vi "CRYTS Sequence Insert.vi"(10 "Steps":refnum<vi>, 11 "Tree Task SequenceIn":refnum<vi>) -> (3 "Tree Task Sequence Out":refnum<vi>)   [LabVIEW 2013]
uses:
  CRYProject Editor Global.vi
  CRYMainGlobal.vi
  CRYCurveLibrary/Global/CRYCurve Library Global.vi
panel:
  # "Insert new step into Project window."
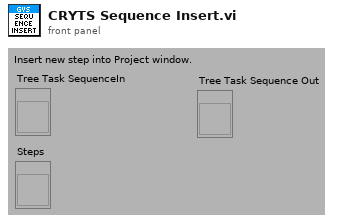
[diagram p1: front panel]
types:
  T1 = typedef "CRYTS.ctl" = cluster{"No.TS":u16, "TS File Path":path, "TS Name":string, "EditStepName":string, "Steps":T2[], "New State":bool, "Change State":bool, "Flattened CurveLib Data":string, "Document Data":string, "EditStepNo":u16, "Operator Start File":string, "Sequence Type":string, "Sequence Language":string}
  T2 = typedef "CRYStep.ctl" = cluster{"No.VI":i32, "Category":string, "StepName":string, "Seq setup flattened":string, "Comment":string, "Steps config.":bool[], "Jump config":i32[], "Start":dbl, "Increment":dbl, "Name":string, "Unit":string, "Y data":u16, "Y prefix":string, "Y dB ref":dbl, "Y unit":string, "Repeat State Array":cluster{"Start":dbl, "Increment":dbl, "Count":i32, "Num":i32}[]}
  T3 = typedef "CRYSequence Cluster.ctl" = cluster{"EditStepName":string, "Trimmed string array":string, "Flattened CurveData":string, "Document Data":string, "EditStepNo":u16, "Operator Start File":path, "Sequence Type":string, "Sequence Language":string, "Sequence Work State":string}
  T4 = cluster{"Data type":string, "Version":u16, "Dimensions":u8}
  T5 = enum32{"English", "Chinese", "Korean", "Japanese", "Russian", "Chinese traditional"}
  T6 = enum16{"OK", "Yes", "YesNo", "YesNoCancel", "ReplaceAppend"}
  T7 = enum16{"Insert", "Remove", "Move up", "Move down"}
  T8 = cluster{"Start":dbl, "Increment":dbl, "Count":i32, "Num":i32}[]
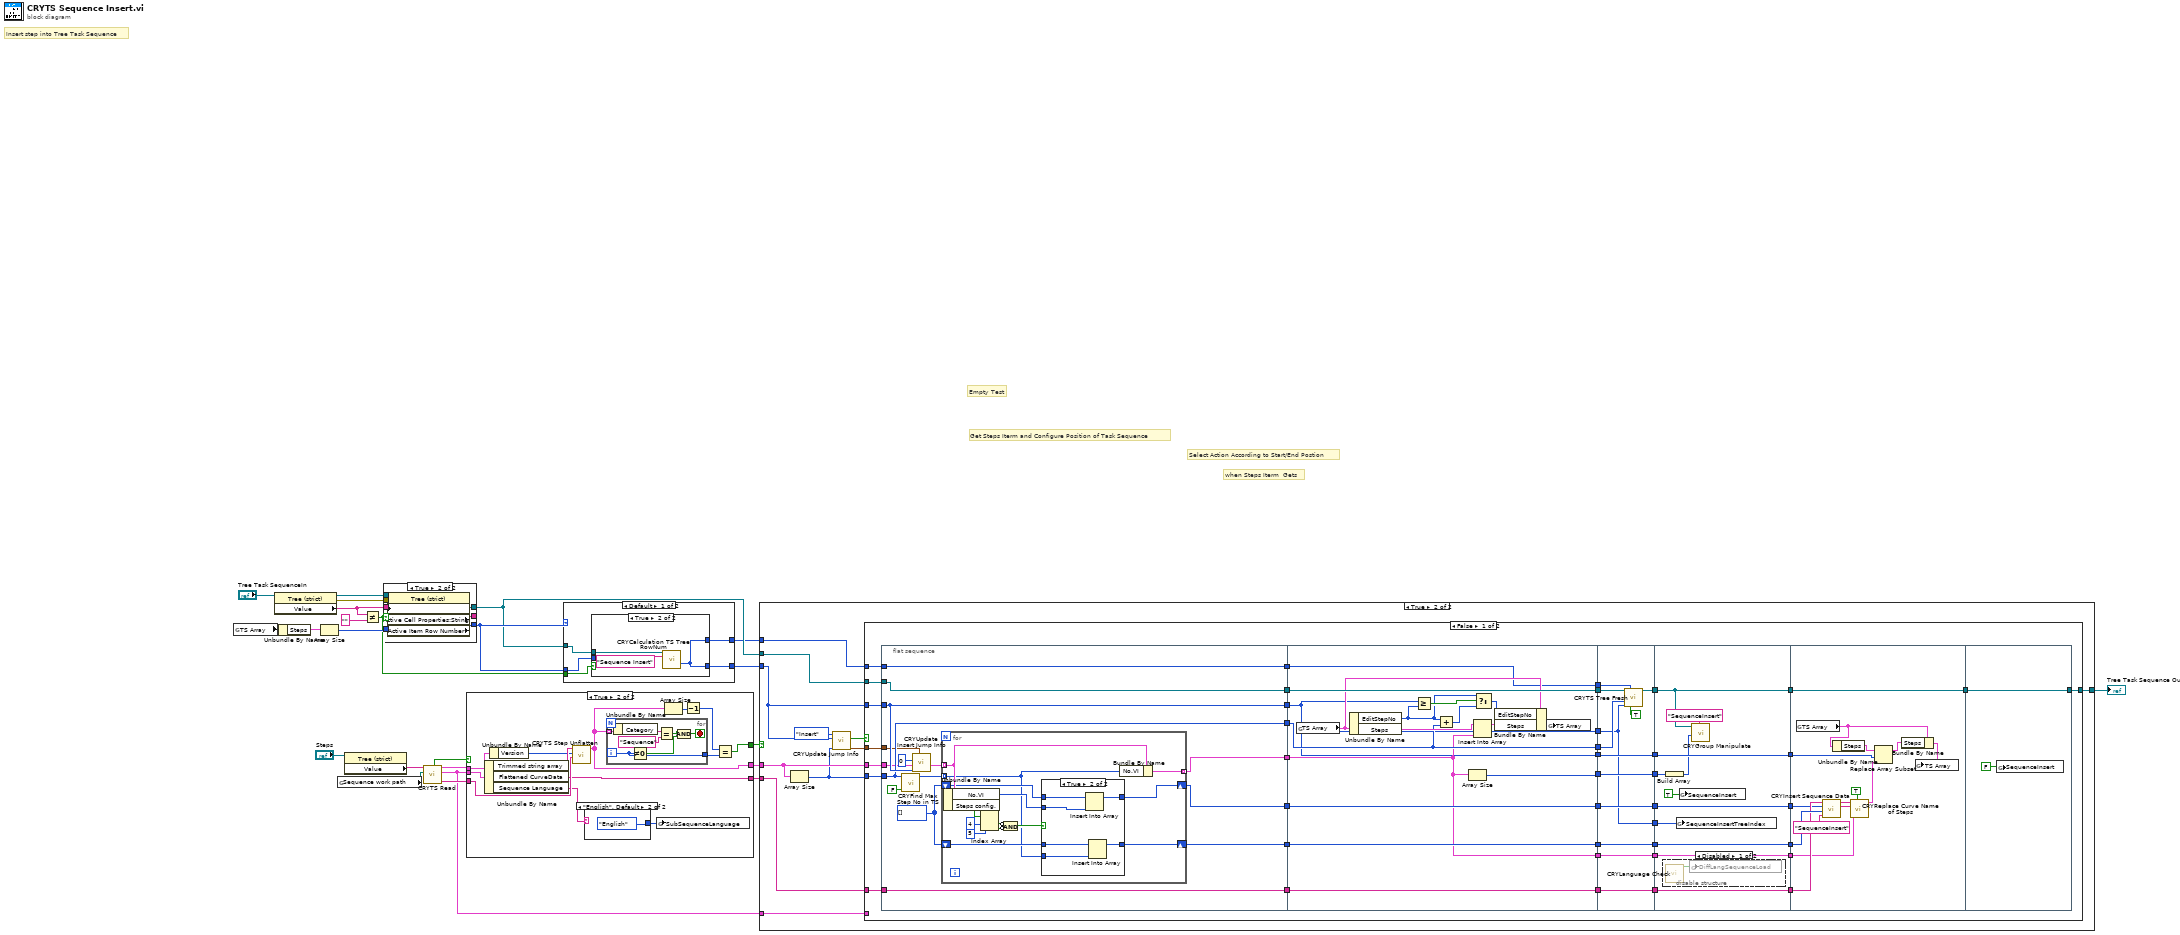
[diagram p0: block diagram]
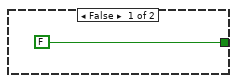
[diagram p2: hidden frame]
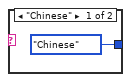
[diagram p3: hidden frame]
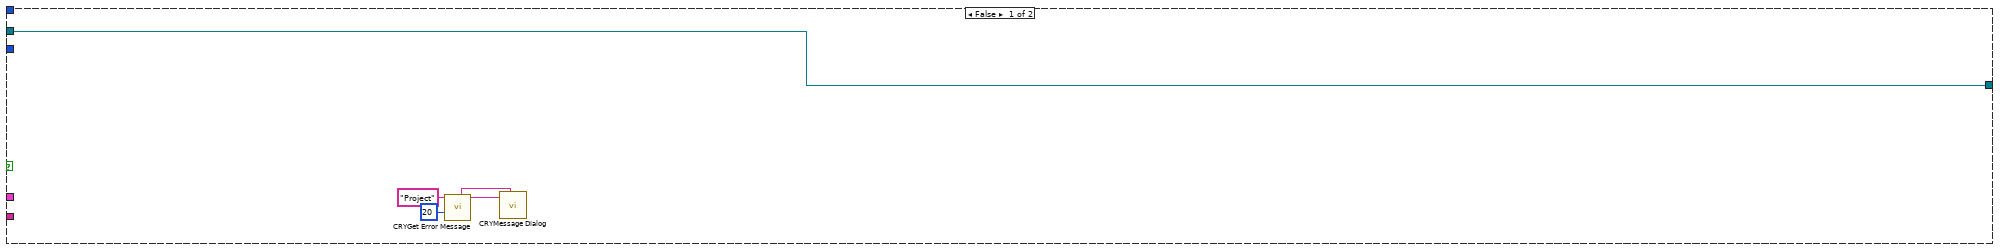
[diagram p4: hidden frame]
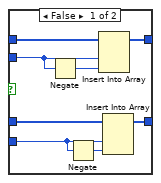
[diagram p5: hidden frame]
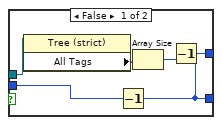
[diagram p8: hidden frame]
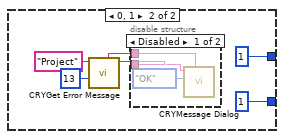
[diagram p9: hidden frame]
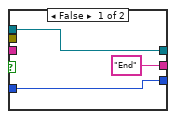
[diagram p11: hidden frame]
diagram:
  # "when Steps Iterm  Gets"
  # "Select Action According to Start/End Postion"
  # "Get Steps Iterm and Configure Position of Task Sequence"
  # "Empty Test"
  # "Insert step into Tree Task Sequence"
  n1 = global read "CRYProject Editor Global.vi" "TS Array"() -> (w22:T1)
  n2 = property class="Tree (strict)"(reference="Tree Task SequenceIn") -> (reference out=w18:refnum<vi>, error out=w17:errorcluster, "Value"=w16:string)  [unwired: 1 in]
  n3 = Unbundle By Name(w22) -> ("Steps"=w19:T2[])
  n4 = Array Size(array=w19) -> (size(s)=w14:i32)
  n5 = global read "CRYMainGlobal.vi" "Sequence work path"() -> (w9:path)
  n6 = property class="Tree (strict)"(reference="Steps") -> ("Value"=w20:string)  [unwired: 1 in, 2 out]
  n7 = Not Equal?(x=w16, y="") -> (x != y?=w6:bool)
  n8 = case shown="True" w6 {
    tunnel: w17 -> [_ w33]
    tunnel: ["End" ("Cell String") w32] -> _
    tunnel: [w25 w31] -> w7
    tunnel: [w27 w30] -> w5
    tunnel: w16 -> [_ w29]
    tunnel: w18 -> [w27 w28]
    tunnel: w14 -> [w25 _]
    frame False {
    }
    frame True {
      n9 = property class="Tree (strict)"(reference=w28, error in=w33, "Active Item Properties:Active Item (Tag)"=w29) -> (reference out=w30:refnum<vi>, "Active Cell Properties:String"=w32:string, "Active Item Row Number"=w31:i32)  [unwired: 1 out]
    }
  }
  n10 = call "CRYTS Read.vi"("Sequence folder path"=w9, "File Name"=w20) -> ("Sequence Name"=w12:string, "sequence list"=w1:T3, "Header info"=w10:T4, "status"=w11:bool)  [unwired: 6 out]
  n11 = case shown="True" w11 {
    tunnel: w1 -> [_ w47]
    tunnel: [FALSE ("status") w37] -> w8
    tunnel: w10 -> [_ w45]
    tunnel: w12 -> [_ w43]
    tunnel: [_ w38] -> w4
    tunnel: [_ w42] -> w3
    frame False {
    }
    frame True {
      n12 = Unbundle By Name(w47) -> ("Trimmed string array"=w46:string, "Flattened CurveData"=w42:string, "Sequence Language"=w35:string)
      n13 = Unbundle By Name(w45) -> ("Version"=w44:u16)
      n14 = call "CRYTS Step Unflatten.vi"("Sequence Name"=w43, "Version"=w44, "Flattened Steps"=w46) -> ("Unflattened Steps"=w38:T2[])  [unwired: 8 out]
      n15 = case shown="\"English\", Default" w35 {
        tunnel: [T5."Chinese" ("Language") T5."English" ("Language")] -> w36
        frame "Chinese" {
        }
        frame "English", Default {
        }
      }
      n16 = for {
        tunnel: w38 -> [w56] mode=indexing
        tunnel: [w50] -> w40
        i -> [w50]
        stop <- w51 stop-if-true
        n17 = Unbundle By Name(w56) -> ("Category"=w55:string)
        n18 = Not Equal To 0?(x=w50) -> (x != 0?=w52:bool)
        n19 = Equal?(x=w55, y="Sequence" ("x")) -> (x = y?=w53:bool)
        n20 = Compound Arithmetic op=AND(w53, w52) -> (w51:bool)
      }
      n21 = global write "CRYProject Editor Global.vi" "SubSequenceLanguage"(w36) -> ()
      n22 = Array Size(array=w38) -> (size(s)=w39:i32)
      n23 = Decrement(x=w39) -> (x-1=w41:i32)
      n24 = Equal?(x=w41, y=w40) -> (x = y?=w37:bool)
    }
  }
  n25 = case shown="Default" w7 {
    tunnel: w7 -> [w59 _]
    tunnel: [w58 1 ("Active Item Row Number")] -> w13
    tunnel: w6 -> [w61 _]
    tunnel: w5 -> [w60 _]
    tunnel: [w57 1 ("TargetRowNum")] -> w2
    frame Default {
      n26 = case shown="True" w61 {
        tunnel: w59 -> [w66 _]
        tunnel: [w62 w67] -> w58
        tunnel: w60 -> [w64 w69]
        tunnel: [w62 w67] -> w57
        frame False {
          n27 = property class="Tree (strict)"(reference=w64) -> ("All Tags"=w65:string[])  [unwired: 1 in, 2 out]
          n28 = Decrement(x=w66) -> (x-1=w62:i32)
          n29 = Array Size(array=w65) -> (size(s)=w63:i32)
          n30 = Decrement(x=w63) -> ()  [unwired: 1 out]
        }
        frame True {
          n31 = call "CRYCalculation TS Tree RowNum.vi"("Tree Task SequenceIn"=w69, "sOption"="Sequence Insert") -> ("TargetRowNum"=w67:i32)  [unwired: 7 in, 6 out]
        }
      }
    }
    frame 0, 1 {
      n32 = call "CRYGet Error Message.vi"("Error No"=13, "Kind"="Project") -> ("Message"=w72:string, "Window Title"=w71:string)  [unwired: 4 in, 4 out]
      n33 = disable-structure shown="Disabled" {
        disable-tunnel: w72 -> [w77 _]
        disable-tunnel: w71 -> [w76 _]
        frame Disabled {
          n34 = call "CRYMessage Dialog.vi"("Window Title"=w76, "YesNoCancel"=T6."OK", "Message Content"=w77) -> ()  [unwired: 7 in, 2 out]
        }
        frame Enabled {
        }
      }
    }
  }
  n35 = case shown="True" w8 {
    tunnel: [w83 w94] -> w24
    tunnel: w13 -> [_ w92]
    tunnel: w5 -> [w83 w93]
    tunnel: w4 -> [_ w90]
    tunnel: w3 -> [_ w87]
    tunnel: w2 -> [_ w86]
    tunnel: w1 -> [_ w84]
    frame False {
      n36 = call "CRYGet Error Message.vi"("Error No"=20, "Kind"="Project") -> ("Message"=w82:string, "Window Title"=w81:string)  [unwired: 4 in, 4 out]
      n37 = call "CRYMessage Dialog.vi"("Window Title"=w81, "Message Content"=w82) -> ()  [unwired: 8 in, 2 out]
    }
    frame True {
      n38 = Array Size(array=w90) -> (size(s)=w89:i32)
      n39 = call "CRYUpdate Jump Info.vi"("SourceCount"=w89, "Step number Selected"=w92, "Action"=T7."Insert") -> ("Jump State Out"=w85:T8, "Canceled?"=w91:bool)  [unwired: 7 in]
      n40 = case shown="False" w91 {
        tunnel: w92 -> [w135 _]
        tunnel: [w134 w237] -> w94
        tunnel: w90 -> [w133 _]
        tunnel: w89 -> [w132 _]
        tunnel: w93 -> [w131 w237]
        tunnel: w87 -> [w130 _]
        tunnel: w86 -> [w124 _]
        tunnel: w85 -> [w120 _]
        tunnel: w84 -> [_ _]
        frame False {
          n41 = flat-sequence {
            tunnel: [w148] -> w129
            tunnel: [w150] -> w128
            tunnel: [w149] -> w127
            tunnel: w130 -> [w137]
            tunnel: w131 -> [w148]
            tunnel: w132 -> [w149]
            tunnel: w133 -> [w147]
            tunnel: w135 -> [w150]
            tunnel: w124 -> [w141]
            tunnel: [w141] -> w123
            tunnel: w120 -> [w140]
            tunnel: [w139] -> w119
            tunnel: [w138] -> w116
            tunnel: [w137] -> w114
            tunnel: [w136] -> w112
            tunnel: w129 -> [w195]
            tunnel: w128 -> [w184]
            tunnel: w127 -> [w186]
            tunnel: [w195] -> w126
            tunnel: [w186] -> w125
            tunnel: w123 -> [w185]
            tunnel: [w185] -> w122
            tunnel: [w184] -> w121
            tunnel: w119 -> [w179]
            tunnel: [w184] -> w118
            tunnel: [w183] -> w117
            tunnel: w116 -> [w183]
            tunnel: [w182] -> w115
            tunnel: w114 -> [w182]
            tunnel: [w181] -> w113
            tunnel: w112 -> [w181]
            tunnel: [w180] -> w101
            tunnel: [w179] -> w97
            tunnel: w126 -> [w205]
            tunnel: w125 -> [w206]
            tunnel: w122 -> [w203]
            tunnel: w121 -> [w197]
            tunnel: [w204] -> w111
            tunnel: [w202] -> w109
            tunnel: w118 -> [w202]
            tunnel: [w201] -> w107
            tunnel: w117 -> [w201]
            tunnel: [w200] -> w105
            tunnel: w115 -> [w200]
            tunnel: [w199] -> w103
            tunnel: w113 -> [w199]
            tunnel: w101 -> [w198]
            tunnel: [w198] -> w100
            tunnel: [w197] -> w99
            tunnel: w97 -> [w196]
            tunnel: [w196] -> w96
            tunnel: w111 -> [w213]
            tunnel: [w213] -> w110
            tunnel: w109 -> [w218]
            tunnel: [w218] -> w108
            tunnel: w107 -> [w217]
            tunnel: [w217] -> w106
            tunnel: w105 -> [w216]
            tunnel: [w216] -> w104
            tunnel: w103 -> [w215]
            tunnel: [w215] -> w102
            tunnel: w100 -> [w212]
            tunnel: w99 -> [w209]
            tunnel: w96 -> [w208]
            tunnel: [w208] -> w95
            tunnel: w110 -> [w234]
            tunnel: w108 -> [w231]
            tunnel: w106 -> [w225]
            tunnel: w104 -> [w224]
            tunnel: w102 -> [w223]
            tunnel: [w234] -> w98
            tunnel: w95 -> [w220]
            tunnel: [w236] -> w134
            tunnel: w98 -> [w236]
            frame #0 {
              w143 = i32[] []
              n42 = call "CRYFind Max Step No in TS.vi"("Inputflg"=FALSE, "Required Count"=w149) -> ("Num Array Out"=w144:i32[])  [unwired: 1 in, 8 out]
              n43 = call "CRYUpdate Insert Jump Info.vi"("Jump State In"=w140, "Count"=w150, "Steps In"=w147, "Step number Selected"=0) -> ("Steps Out"=w145:T2[])  [unwired: 6 in, 1 out]
              n44 = for {
                tunnel: w145 -> [w163] mode=indexing
                tunnel: w144 -> [w151] mode=indexing
                tunnel: [w164] -> w139 mode=indexing
                shift-right: [w154] -> w136
                shift-left: w143 -> [w155]
                shift-right: [w152] -> w138
                shift-left: w143 -> [w153]
                n45 = Unbundle By Name(w163) -> ("No.VI"=w156:i32, "Steps config."=w162:bool[])
                n46 = Index Array(array=w162, index #1=4 ("index"), index #2=5 ("index")) -> (element #1=w159:bool, element #2=w158:bool)
                n47 = Compound Arithmetic op=AND(invert w159, invert w158) -> (w157:bool)
                n48 = case shown="True" w157 {
                  tunnel: w156 -> [w170 w176]
                  tunnel: [w171 w177] -> w154
                  tunnel: w155 -> [w172 w178]
                  tunnel: w153 -> [w168 w175]
                  tunnel: [w167 w174] -> w152
                  tunnel: w151 -> [w166 w173]
                  frame False {
                    n49 = Negate(x=w170) -> (-x=w169:i32)
                    n50 = Negate(x=w166) -> (-x=w165:i32)
                    n51 = Insert Into Array(array=w172, new element #1=w170, new element #2=w169) -> (w171:i32[])  [unwired: 1 in]
                    n52 = Insert Into Array(array=w168, new element #1=w166, new element #2=w165) -> (w167:i32[])  [unwired: 1 in]
                  }
                  frame True {
                    n53 = Insert Into Array(array=w178, new element=w176) -> (w177:i32[])  [unwired: 1 in]
                    n54 = Insert Into Array(array=w175, new element=w173) -> (w174:i32[])  [unwired: 1 in]
                  }
                }
                n55 = Bundle By Name(cluster=w163, "No.VI"=w151) -> (w164:T2)
              }
            }
            frame #1 {
              n56 = global read "CRYProject Editor Global.vi" "TS Array"() -> (w191:T1)
              n57 = Unbundle By Name(w191) -> ("EditStepNo"=w188:u16, "Steps"=w190:T2[])
              n58 = Greater Or Equal?(x=w184, y=w188) -> (x >= y?=w189:bool)
              n59 = Add(x=w188, y=w186) -> (x+y=w187:i32)
              n60 = Array Size(array=w179) -> (size(s)=w180:i32)
              n61 = Insert Into Array(array=w190, index=w184, new element=w179) -> (w193:T2[])
              n62 = Select(t=w188, s=w189, f=w187) -> (s? t:f=w194:i32)
              n63 = Bundle By Name(cluster=w191, "EditStepNo"=w194, "Steps"=w193) -> (w192:T1)
              n64 = global write "CRYProject Editor Global.vi" "TS Array"(w192) -> ()
            }
            frame #2 {
              n65 = call "CRYTS Tree Fresh.vi"("SequenceTree"=w205, "Edit Index"=w203, "SourceCount"=w206, "Target Index"=w197, "Is Refresh?"=TRUE) -> ("SequenceTree out"=w204:refnum<vi>)  [unwired: 10 in]
            }
            frame #3 {
              n66 = disable-structure shown="Disabled" {
                frame Disabled {
                  n67 = call "CRYLanguage Check.vi"() -> ("DiffLanguage"=w219:bool)  [unwired: 10 in, 1 out]
                  n68 = global write "CRYCurve Library Global.vi" "DiffLangSequenceLoad"(w219) -> ()
                }
                frame Enabled {
                }
              }
              n69 = Build Array(w212) -> (w211:i32[])
              n70 = global write "CRYProject Editor Global.vi" "SequenceInsertTreeIndex"(w209) -> ()
              n71 = global write "CRYProject Editor Global.vi" "SequenceInsert"(TRUE ("SequenceInsert")) -> ()
              n72 = call "CRYGroup Manipulate.vi"("sAction"="SequenceInsert", "nData"=w211, "Tree in"=w213) -> ()  [unwired: 5 in, 4 out]
            }
            frame #4 {
              n73 = global read "CRYProject Editor Global.vi" "TS Array"() -> (w233:T1)
              n74 = call "CRYInsert Sequence Data.vi"("sOption"="SequenceInsert" ("sAction"), "New Step No."=w225, "Old Step No."=w223, "sFlattenedCurveData"=w224) -> ("New Names Out"=w226:string[], "Old Names Out"=w227:string[])  [unwired: 6 in]
              n75 = Unbundle By Name(w233) -> ("Steps"=w232:T2[])
              n76 = call "CRYReplace Curve Name of Steps.vi"("Option flg"=TRUE, "Steps In"=w220, "New Name"=w226, "Old Name"=w227) -> ("Steps Out"=w222:T2[])  [unwired: 7 in]
              n77 = Replace Array Subset(array=w232, new element=w222, index=w231) -> (w230:T2[])
              n78 = Bundle By Name(cluster=w233, "Steps"=w230) -> (w229:T1)
              n79 = global write "CRYProject Editor Global.vi" "TS Array"(w229) -> ()
            }
            frame #5 {
              n80 = global write "CRYProject Editor Global.vi" "SequenceInsert"(FALSE ("SequenceInsert")) -> ()
            }
          }
        }
        frame True {
        }
      }
    }
  }
  "Tree Task Sequence Out" <- w24
